vi "Find Control.vi"() -> ()   [LabVIEW 2015]
doc: "Example VI that demonstrates finding control in VI and cluster."
uses:
  PL Utility.lvlib
panel:
  in  "cluster":cluster{"control":i32}
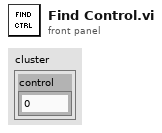
[diagram p1: front panel]
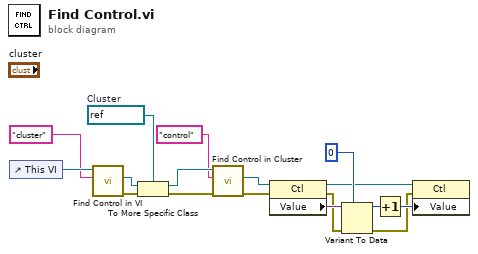
[diagram p0: block diagram]
diagram:
  w14 = refnum<vi> refnum  # Cluster
  n1 = control-ref of="This VI"() -> (w17:refnum<vi>)
  n2 = call "Find Control in VI.vi"("control label"="cluster", "vi reference in"=w17) -> ("error out"=w16:errorcluster, "control reference"=w15:refnum<vi>)  [unwired: 7 in, 1 out]
  n3 = To More Specific Class(target class=w14, reference=w15, error in=w16) -> (specific class reference=w12:refnum<vi>, error out=w13:errorcluster)
  n4 = call "Find Control in Cluster.vi"("error in (no error)"=w13, "control label"="control", "cluster reference in"=w12) -> ("error out"=w8:errorcluster, "control reference"=w9:refnum<vi>)  [unwired: 6 in, 1 out]
  n5 = property class="Ctl"(reference=w9, error in=w8) -> (reference out=w4:refnum<vi>, error out=w6:errorcluster, "Value"=w7:variant)
  n6 = Variant To Data(error in=w6, type=0 ("control"), Variant=w7) -> (data=w3:i32, error out=w1:errorcluster)
  n7 = Increment(x=w3) -> (x+1=w2:i32)
  n8 = property class="Ctl"(reference=w4, error in=w1, "Value"=w2) -> ()  [unwired: 2 out]
